vi "Marker Out Spreading.vi"   [LabVIEW 2014, in "Wavepond.lvclass"]
uses:
  Wavepond.lvclass
  <vilib>/DAQmx/create/channels.llb/DAQmx Create Channel (CO-Pulse Generation-Ticks).vi
  <vilib>/DAQmx/configure/trigger.llb/DAQmx Start Trigger (Digital Edge).vi
  <resource>/objmgr/daqmx.rc
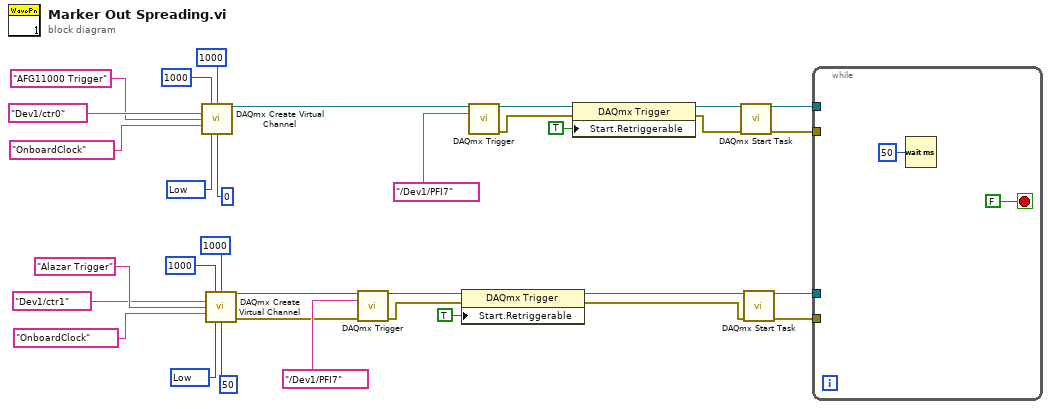
[diagram p0: block diagram]
diagram:
  w12 = 10214 items=["High"=10192, "Low"=10214] ("idle state")
  w32 = 10214 items=["High"=10192, "Low"=10214] ("idle state")
  n1 = call-poly <vilib>:"DAQmx Create Virtual Channel.vi"("high ticks"=u32 1000, "low ticks"=u32 1000, "counter"=tag "Dev1/ctr0", "name to assign"="AFG11000 Trigger", "source of ticks"=tag "OnboardClock", "idle state"=w32, "initial delay"=u32 0) -> ("task out"=w20:refnum<k21>)  [unwired: 7 in, 1 out]
  n2 = call-poly <vilib>:"DAQmx Create Virtual Channel.vi"("high ticks"=u32 1000, "low ticks"=u32 1000, "counter"=tag "Dev1/ctr1", "name to assign"="Alazar Trigger", "source of ticks"=tag "OnboardClock", "idle state"=w12, "initial delay"=u32 50) -> ("task out"=w5:refnum<k21>, "error out"=w6:errorcluster)  [unwired: 7 in]
  n3 = call-poly <vilib>:"DAQmx Trigger.vi"("task/channels in"=w5, "source"=tag "/Dev1/PFI7" ("source of ticks"), "error in"=w6) -> ("task out"=w8:refnum<k21>, "error out"=w10:errorcluster)  [unwired: 11 in]
  n4 = property class="DAQmx Trigger"(reference=w8, error in=w10, "Start.Retriggerable"=TRUE) -> (reference out=w4:refnum<k21>, error out=w3:errorcluster)
  n5 = call-poly <vilib>:"DAQmx Trigger.vi"("task/channels in"=w20, "source"=tag "/Dev1/PFI7" ("source of ticks")) -> ("task out"=w25:refnum<k21>, "error out"=w22:errorcluster)  [unwired: 12 in]
  n6 = property class="DAQmx Trigger"(reference=w25, error in=w22, "Start.Retriggerable"=TRUE) -> (reference out=w23:refnum<k21>, error out=w21:errorcluster)
  n7 = call <vilib>:"DAQmx Start Task.vi"("task/channels in"=w23, "error in"=w21) -> ("task out"=w18:refnum<k21>, "error out"=w19:errorcluster)  [unwired: 12 in]
  n8 = call <vilib>:"DAQmx Start Task.vi"("task/channels in"=w4, "error in"=w3) -> ("task out"=w2:refnum<k21>, "error out"=w1:errorcluster)  [unwired: 12 in]
  n9 = while {
    tunnel: w19 -> [_]
    tunnel: w18 -> [_]
    tunnel: w2 -> [_]
    tunnel: w1 -> [_]
    stop <- FALSE stop-if-true
    n10 = Wait (ms)(milliseconds to wait=u32 50) -> ()  [unwired: 1 out]
  }
